vi "tmp2bindata to flat.vi"(7 "type in":i64, 8 "error in (no error)":errorcluster, 9 "start":i32=-1, 10 "nofbytes":i32=-1, 11 "bindata in":u8[](array[numeric])) -> (0 "error out":errorcluster, 2 "x-y*floor(x/y)":i32, 3 "numarray out":i64[](array[numeric]))   [LabVIEW 2018]
uses:
  <vilib>/Utility/error.llb/Error Cluster From Error Code.vi
  <vilib>/ErrorRing/Error Ring.xnode
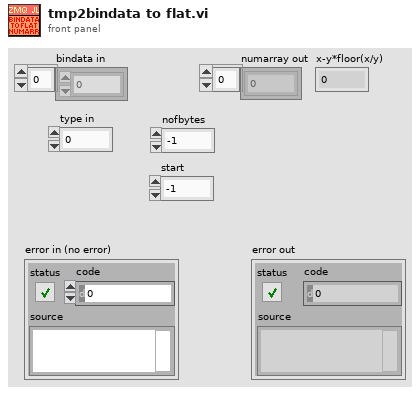
[diagram p1: front panel]
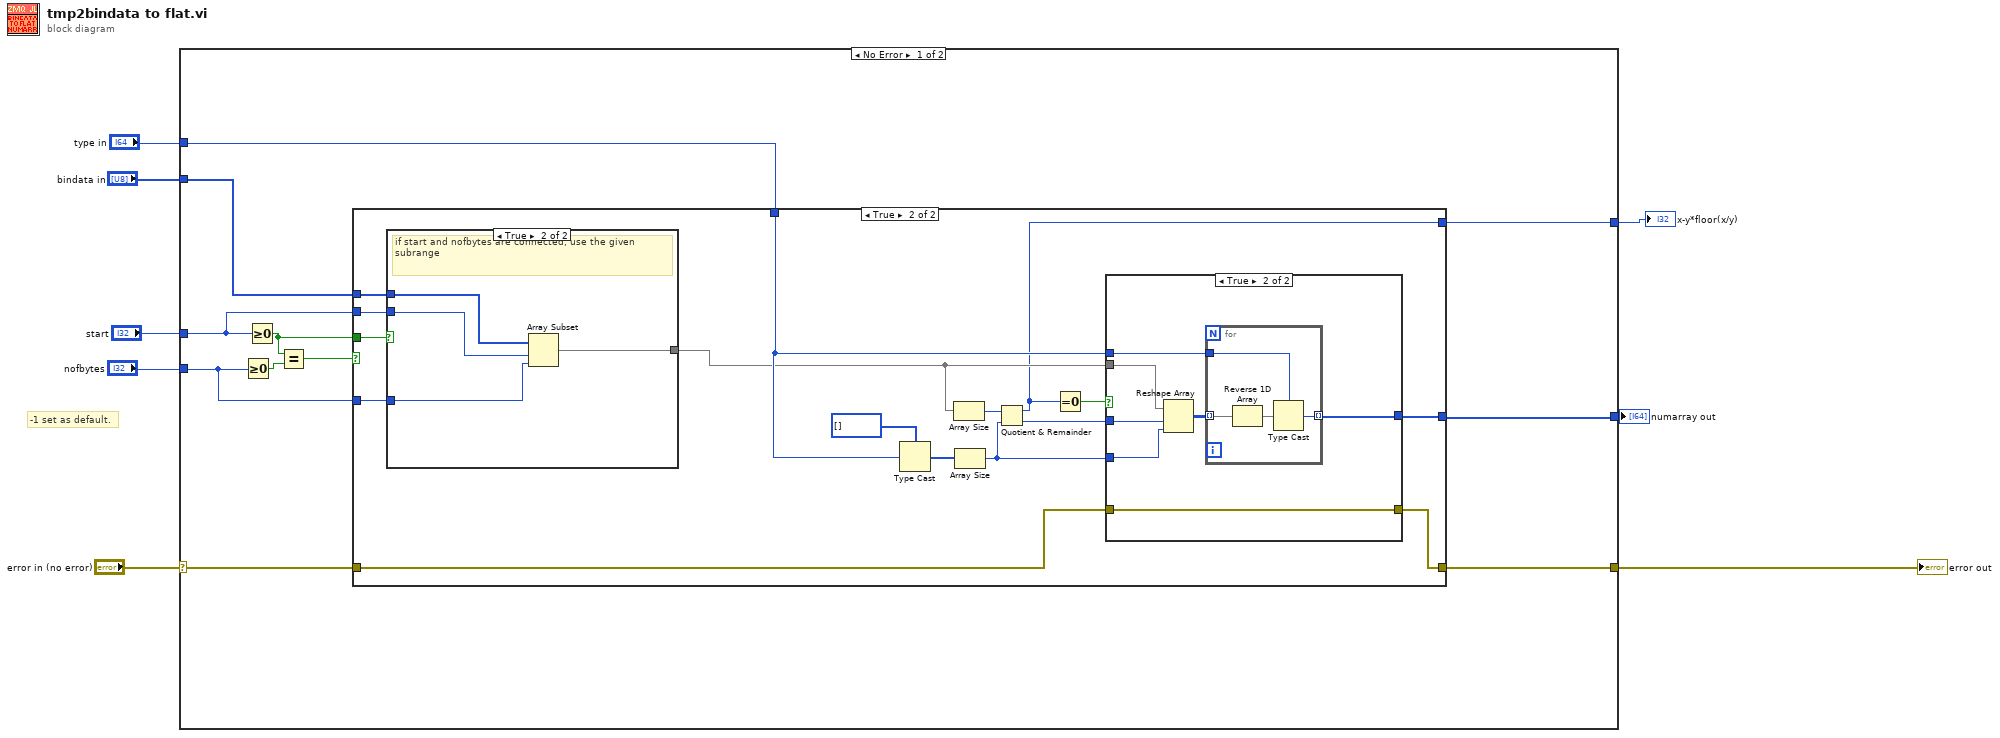
[diagram p0: block diagram]
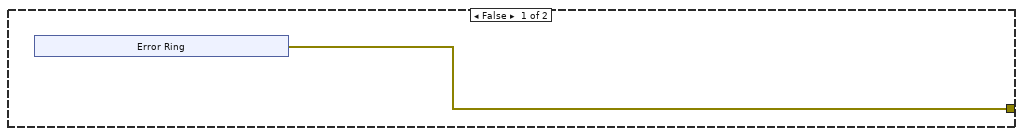
[diagram p2: hidden frame]
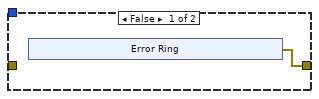
[diagram p3: hidden frame]
diagram:
  # "-1 set as default."
  n1 = case shown="No Error" "error in (no error)" {
    selector: "error in (no error)" -> [w17 w64]
    tunnel: [w10 _] -> w8
    tunnel: "bindata in" -> [w15 _]
    tunnel: "type in" -> [w11 _]
    tunnel: "nofbytes" -> [w13 _]
    tunnel: "start" -> [w14 _]
    tunnel: [w18 w64] -> w2
    tunnel: [w9 _] -> w1
    frame No Error {
      n2 = Greater Or Equal To 0?(x=w13) -> (x >= 0?=w16:bool)
      n3 = Greater Or Equal To 0?(x=w14) -> (x >= 0?=w12:bool)
      n4 = Equal?(x=w12, y=w16) -> (x = y?=w19:bool)
      n5 = case shown="True" w19 {
        tunnel: [w20 w27] -> w18
        tunnel: w17 -> [_ w28]
        tunnel: w15 -> [_ w41]
        tunnel: w14 -> [_ w40]
        tunnel: w13 -> [_ w39]
        tunnel: w12 -> [_ w38]
        tunnel: w11 -> [_ w32]
        tunnel: [_ w30] -> w10
        tunnel: [_ w26] -> w9
        frame False {
          n6 = xnode "Error Ring"() -> ("error out"=w20:errorcluster)
        }
        frame True {
          n7 = case shown="True" w38 {
            tunnel: w41 -> [w59 w63]
            tunnel: w40 -> [_ w62]
            tunnel: w39 -> [_ w61]
            tunnel: [w59 w60] -> w31
            frame False {
              # "for default start&nofbytes values, use the full bindata range"
            }
            frame True {
              # "if start and nofbytes are connected, use the given subrange"
              n8 = Array Subset(array=w63, index=w62, length=w61) -> (w60:u8[])
            }
          }
          n9 = Type Cast(type=u8[] [] ("bindata in"), x=w32) -> (*(type *) &x=w34:u8[])
          n10 = Array Size(array=w31) -> (size(s)=w35:i32)
          n11 = Array Size(array=w34) -> (size(s)=w37:i32)
          n12 = Quotient & Remainder(x=w35, y=w37) -> (x-y*floor(x/y)=w26:i32, floor(x/y)=w36:i32)
          n13 = Equal To 0?(x=w26) -> (x = 0?=w29:bool)
          n14 = case shown="True" w29 {
            tunnel: w37 -> [_ w53]
            tunnel: w36 -> [_ w52]
            tunnel: w32 -> [_ w51]
            tunnel: w31 -> [_ w50]
            tunnel: [_ w49] -> w30
            tunnel: [w42 w48] -> w27
            tunnel: w28 -> [_ w48]
            frame False {
              n15 = xnode "Error Ring"() -> ("error out"=w42:errorcluster)
            }
            frame True {
              n16 = Reshape Array(w50, w52, w53) -> (w54:u8[][])
              n17 = for {
                tunnel: w54 -> [w58] mode=indexing
                tunnel: w51 -> [w56]
                tunnel: [w55] -> w49 mode=indexing
                n18 = Reverse 1D Array(array=w58) -> (reversed array=w57:u8[])
                n19 = Type Cast(type=w56, x=w57) -> (*(type *) &x=w55:i64)
              }
            }
          }
        }
      }
    }
    frame Error {
    }
  }
  "numarray out" <- w8
  "error out" <- w2
  "x-y*floor(x/y)" <- w1
